vi "Initialize Lidar.vi"(8 "error in (no error)":errorcluster) -> (0 "error out":errorcluster, 3 "SerialPortRef":T1)   [LabVIEW 2013]
uses:
  <vilib>/Rock Robotics/WPI/SerialPort/WPI_SerialPortRef.ctl
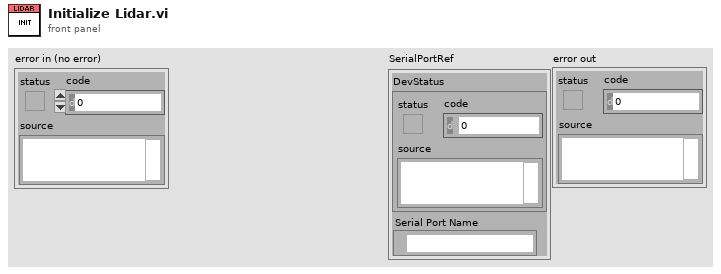
[diagram p1: front panel]
types:
  T1 = typedef "WPI_SerialPortRef.ctl" = cluster{"DevStatus":errorcluster, "Serial Port Name":refnum<visa-resource-name>}
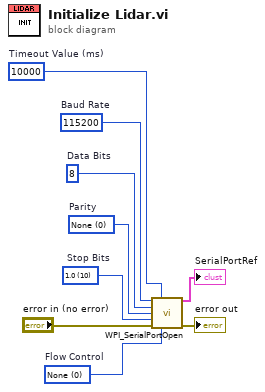
[diagram p0: block diagram]
diagram:
  w4 = u32 10000  # Timeout Value (ms)
  w5 = u16 0 items=["None", "XON/XOFF", "RTS/CTS", "XON/XOFF & RTS/CTS", "DTR/DSR", "XON/XOFF & DTR/DSR"]  # Flow Control
  w6 = u16 10 items=["1.0"=10, "1.5"=15, "2.0"=20]  # Stop Bits
  w7 = u16 0 items=["None", "Odd", "Even", "Mark", "Space"]  # Parity
  w8 = u16 8  # Data Bits
  w9 = u32 115200  # Baud Rate
  n1 = call <vilib>:"WPI_SerialPortOpen.vi"("Baud Rate"=w9, "Timeout Value (ms)"=w4, "Data Bits"=w8, "Parity"=w7, "Stop Bits"=w6, "error in (no error)"="error in (no error)", "Flow Control"=w5) -> ("SerialPortRef"=→"SerialPortRef":T1, "error out"=→"error out":errorcluster)  [unwired: 7 in]
